vi "DIO 8-bit.vi"(0 "DIO 7 Refnum":refnum<k21>, 3 "DIO 0 Refnum":refnum<k21>, 4 "DIO 6 Refnum":refnum<k21>, 5 "DIO 1 Refnum":refnum<k21>, 6 "DIO 5 Refnum":refnum<k21>, 7 "DIO 2 Refnum":refnum<k21>, 8 "DIO 4 Refnum":refnum<k21>, 9 "DIR 7:0":u8 format="%08b", 10 "OUT 7:0":u8 format="%08b", 11 "DIO 3 Refnum":refnum<k21>) -> (2 "IN 7:0":u8 format="%08b")   [LabVIEW 2014]
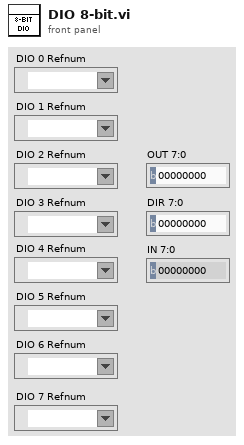
[diagram p1: front panel]
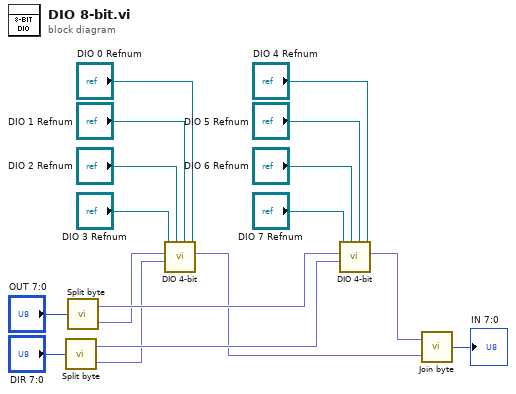
[diagram p0: block diagram]
diagram:
  n1 = call "Split byte.vi"("x"="DIR 7:0") -> ("hi(x)"=w5:fxp<+,4,4>, "lo(x)"=w3:fxp<+,4,4>)
  n2 = call "Split byte.vi"("x"="OUT 7:0") -> ("hi(x)"=w6:fxp<+,4,4>, "lo(x)"=w4:fxp<+,4,4>)
  n3 = call "DIO 4-bit.vi"("DIO0 Refnum"="DIO 0 Refnum", "DIO1 Refnum"="DIO 1 Refnum", "DIO2 Refnum"="DIO 2 Refnum", "DIR 3:0"=w3, "OUT 3:0"=w4, "DIO3 Refnum"="DIO 3 Refnum") -> ("IN 3:0"=w1:fxp<+,4,4>)  [unwired: 5 in]
  n4 = call "DIO 4-bit.vi"("DIO0 Refnum"="DIO 4 Refnum", "DIO1 Refnum"="DIO 5 Refnum", "DIO2 Refnum"="DIO 6 Refnum", "DIR 3:0"=w5, "OUT 3:0"=w6, "DIO3 Refnum"="DIO 7 Refnum") -> ("IN 3:0"=w2:fxp<+,4,4>)  [unwired: 5 in]
  n5 = call "Join byte.vi"("lo"=w1, "hi"=w2) -> ("hi.lo"=→"IN 7:0":u8)
